vi "CopyFIFO.vi"(0 "Input":refnum<k21>) -> ()   [LabVIEW 2018]
uses:
  <vilib>/rvi/DataTransferAndStorage/Container/Common/niFpgaContainerExecOnDevCompGetState.vi
  <vilib>/rvi/Emulation/niFpgaEmulationIsFPGAContextNoSignature.vi
  <vilib>/rvi/Emulation/niFpgaSctlEmulationGetInTimedLoop.vi
  <vilib>/rvi/errors/niFpgaSetErrorForExecOnDevCompSimple.vi
  <vilib>/rvi/eio/common/nirviEmuReportErrorAndStop.vi
  <vilib>/rvi/DataTransferAndStorage/Container/Common/niFpgaContainerGetUniqueNameForEmu.vi
  <vilib>/rvi/FIFO/Fifo_Resource/nirvififoEmulationSetSize.vi
  <vilib>/rvi/FIFO/Fifo_Resource/nirviFifoEmulationQueueMgr.vi
  <instcachedir>/0/nirviFifoEmulationQueueMgr_E5CAEC123FF24DC58D834DCA3CDAA9B5.lvgen/nirviFifoEmulationQueueMgr_E5CAEC123FF24DC58D834DCA3CDAA9B5_001.vi
  <vilib>/rvi/FIFO/Fifo_Resource/nirvififoEmulationDetermineInputValidOut.vi
  <vilib>/rvi/FIFO/Fifo_Resource/nirvififoEmulationCreateLock.vi
  <vilib>/rvi/Emulation/niFpgaProcessEmulError.vi
  <vilib>/rvi/FIFO/Fifo_Resource/nirvififoEmulationObtainLock.vi
  <vilib>/rvi/FIFO/Fifo_Resource/nirvififoEmulationReleaseLock.vi
  <vilib>/rvi/occurrence/nirviWaitOnOccurrenceBase.vi
  <vilib>/rvi/errors/nirviReportUnexpectedCaseInternalError.vi
  <vilib>/rvi/errors/nirviReportUnexpectedCaseInternalError (U32).vi
  <vilib>/Utility/error.llb/Clear Errors.vi
  <vilib>/rvi/interface/RandomDataEmulation/niFpgaRandomDataHandleErrors.vi
  <vilib>/rvi/DataTransferAndStorage/Container/XNode/niFpgaContainer.xnode
  <vilib>/rvi/FIFO/Fifo_Resource/niFpgaFifoEmulationRefIn.vi
  <vilib>/rvi/interface/RandomDataEmulation/nirviRandomDataFpgaReadWriteTemplate.vi
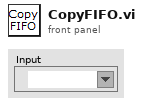
[diagram p1: front panel]
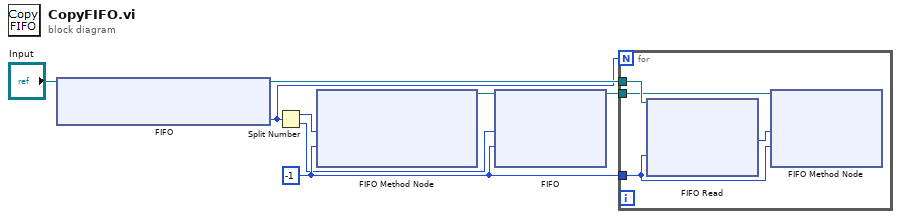
[diagram p0: block diagram]
diagram:
  w2 = -1 ("Timeout")
  n1 = xnode "FIFO"("FIFO In"="Input") -> ("Number of Elements to Read"=w6:u32, "FIFO Out"=w7:refnum<k21>)
  n2 = Split Number(x=w6) -> (hi(x)=w4:u16, lo(x)=w1:u16)
  n3 = xnode ("FIFO Method Node")("Element"=w4, "Timeout"=w2) -> ("FIFO Out"=w5:refnum<k21>)  [unwired: 1 in, 1 out]
  n4 = xnode "FIFO"("Element"=w1, "Timeout"=w2, "FIFO In"=w5) -> ("FIFO Out"=w3:refnum<k21>)  [unwired: 1 out]
  n5 = for {
    N: w6 -> [_]
    tunnel: w2 -> [w12]
    tunnel: w7 -> [w11]
    tunnel: w3 -> [w9]
    n6 = xnode ("FIFO Read")("Timeout"=w12, "FIFO In"=w11) -> ("Element"=w10:u8)  [unwired: 2 out]
    n7 = xnode ("FIFO Method Node")("Element"=w10, "Timeout"=w12, "FIFO In"=w9) -> ()  [unwired: 2 out]
  }
